vi "Auto Find ConfigFile Folder.vi"(10 "ConfigFile":string="ConfigFile", 11 "Application Directory":path) -> (3 "Project Folder":path)   [LabVIEW 2021, in "TopPath.lvlib"]
doc: "auto find Project Main Folder"
uses:
  TopPath.lvlib
panel:
  out "Array":path[](array[path])
  out "folder names":string[](array[string])
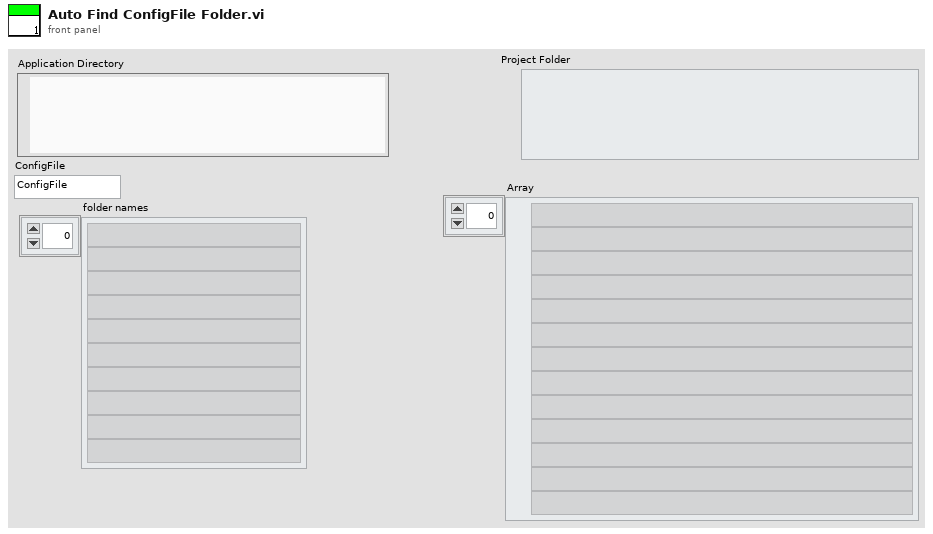
[diagram p1: front panel]
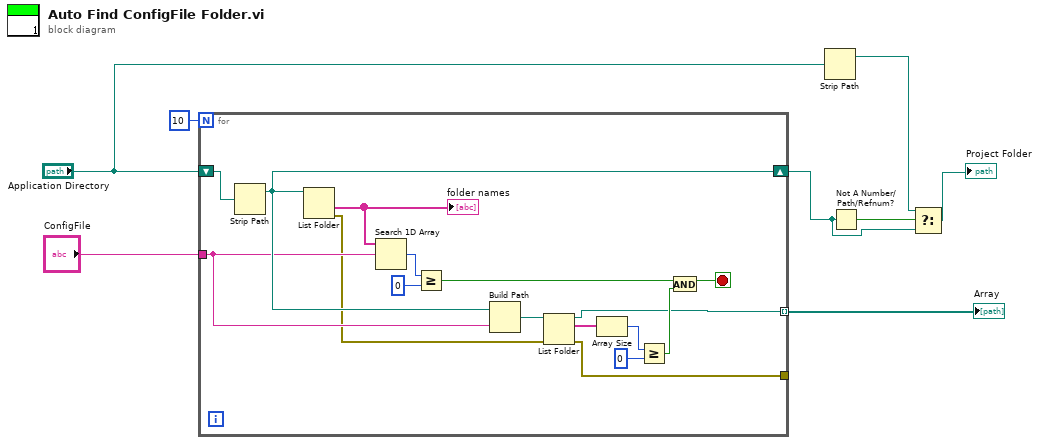
[diagram p0: block diagram]
diagram:
  n1 = for {
    N: 10 -> [_]
    shift-right: [w19] -> w2
    shift-left: "Application Directory" -> [w24]
    tunnel: "ConfigFile" -> [w18]
    tunnel: [w11] -> w6 mode=indexing
    tunnel: [w10] -> _
    stop <- w13 stop-if-true
    n2 = Strip Path(path=w24) -> (stripped path=w19:path)  [unwired: 1 out]
    n3 = List Folder(path=w19) -> (folder names=w23:string[], error out=w9:errorcluster)  [unwired: 3 in, 2 out]
    "folder names" <- w23
    n4 = Search 1D Array(1D array=w23, element=w18) -> (index of element=w22:i32)  [unwired: 1 in]
    n5 = Greater Or Equal?(x=w22, y=0) -> (x >= y?=w20:bool)
    n6 = Build Path(base path=w19, name or relative path=w18) -> (appended path=w17:path)
    n7 = List Folder(path=w17, error in=w9) -> (path out=w11:path, filenames=w16:string[], error out=w10:errorcluster)  [unwired: 2 in, 1 out]
    n8 = Array Size(array=w16) -> (size(s)=w15:i32)
    n9 = Greater Or Equal?(x=w15, y=0) -> (x >= y?=w12:bool)
    n10 = And(x=w20, y=w12) -> (x .and. y?=w13:bool)
  }
  "Array" <- w6
  n11 = Strip Path(path="Application Directory") -> (stripped path=w3:path)  [unwired: 1 out]
  n12 = Not A Number/Path/Refnum?(number/path/refnum=w2) -> (NaN/Path/Refnum?=w4:bool)
  n13 = Select(t=w3, s=w4, f=w2) -> (s? t:f=→"Project Folder":path)
